vi "Type Info.vi"(11 "Build Package Item in":refnum<class "Build Package Item.lvclass">) -> (1 "Description":string, 2 "Pretty Name":string, 3 "Type":string)   [LabVIEW 2019, in "VIPM.lvlib" / "Build Package Item.lvclass"]
doc: "Returns Type information about the solution item.\n----\nCopyright: MGI 2017\nAuthor: Derek Trepanier"
uses:
  Build Package Item.lvclass
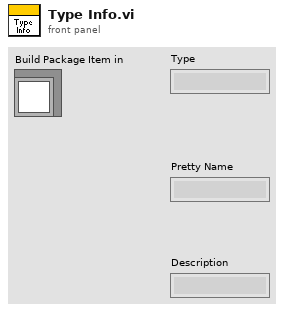
[diagram p1: front panel]
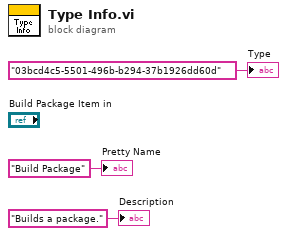
[diagram p0: block diagram]
diagram:
  "Pretty Name" <- "Build Package" ("Pretty Name")
  "Description" <- "Builds a package." ("Description")
  "Type" <- "03bcd4c5-5501-496b-b294-37b1926dd60d" ("Type")
